vi "CRYAPI Temp Frame.vi"() -> ()   [LabVIEW 2013]
uses:
  <vilib>/Utility/miscctls.llb/LVPointTypeDef.ctl
  <vilib>/Utility/miscctls.llb/LVPositionTypeDef.ctl
  <vilib>/Utility/miscctls.llb/LVBoundsTypeDef.ctl
  <vilib>/Utility/inputDevices.llb/closeMouse.vi
  CRYMain Sub Window Global.vi
  <vilib>/Utility/inputDevices.llb/mouseAcquire.vi
panel:
  in  "StateOut":bool
  in  "IconRing":u16(ring)
  out "bTitleChange":bool
  in  "WindowNumber":i32=2
  in  "ActiveNumber":i32=2
  out "TitleName":string="Project"
  in  "PinFalse":bool
  in  "PinTrue":bool
  in  "stop":bool
  in  "InActiveClose":bool
  in  "ActiveClose":bool
  in  "nWinType":i32=2
  in  "MousePos":T1
  in  "sMsgCommand":string="Project"
  in  "nData":i32=2
  in  "FloatEvent":bool
  out "SubVI Ref":refnum<vi>
  in  "WindowName":string="Project"
  in  "DockState":bool
  in  "ActiveState":bool
  in  "ToolBarClick":bool
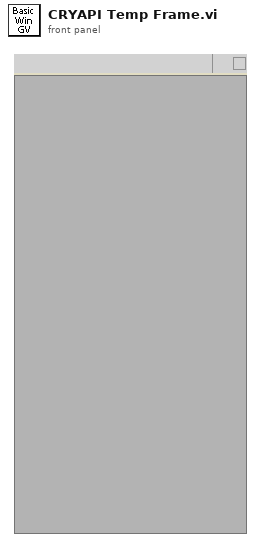
[diagram p1: front panel]
types:
  T1 = cluster{"Horizontal":i32, "Vertical":i32, "Scrolling":i32}
  T2 = typedef "LVBoundsTypeDef.ctl" = cluster{"Width":u32, "Height":u32}
  T3 = typedef "LVPositionTypeDef.ctl" = cluster{"Left":i32, "Top":i32}
  T4 = typedef "LVPointTypeDef.ctl" = cluster{"Horizontal":i16, "Vertical":i16}
  T5 = typedef "LVRectTypeDef.ctl" = cluster{"Left":i16, "Top":i16, "Right":i16, "Bottom":i16}
  T6 = cluster{"button 1":bool, "button 2":bool, "button 3":bool, "button 4":bool}
  T7 = cluster{"CLOSE_HIDE":i32, "CLOSE_CLOSE":i32, "DOCK_ENABLE":i32, "DOCK_DISABLE":i32, "FOCUS_SHOW":i32, "FOCUS_HIDE":i32}
  T8 = cluster{"nType":i32, "nParent":i32, "pVIW":refnum<vi>, "pSPW":refnum<vi>, "nTypeF":i32, "pVIF":refnum<vi>, "pSPF":refnum<vi>, "nIDSpliter":i32, "nProperty":i32, "Bound":T5, "nID":i32, "nData":i32, "sData":string, "pWVI":refnum<vi>, "sTitle":string, "cPages":cluster{"nPage":i32, "sTitle":string, "sIcon":string, "pVI":refnum<vi>, "nID":i32}[], "pTab":refnum<vi>, "nIDPages":i32[], "pSPT":refnum<vi>, "sTemp":string, "nDockID":i32, "nDockLR":i32, "sIcon":string}
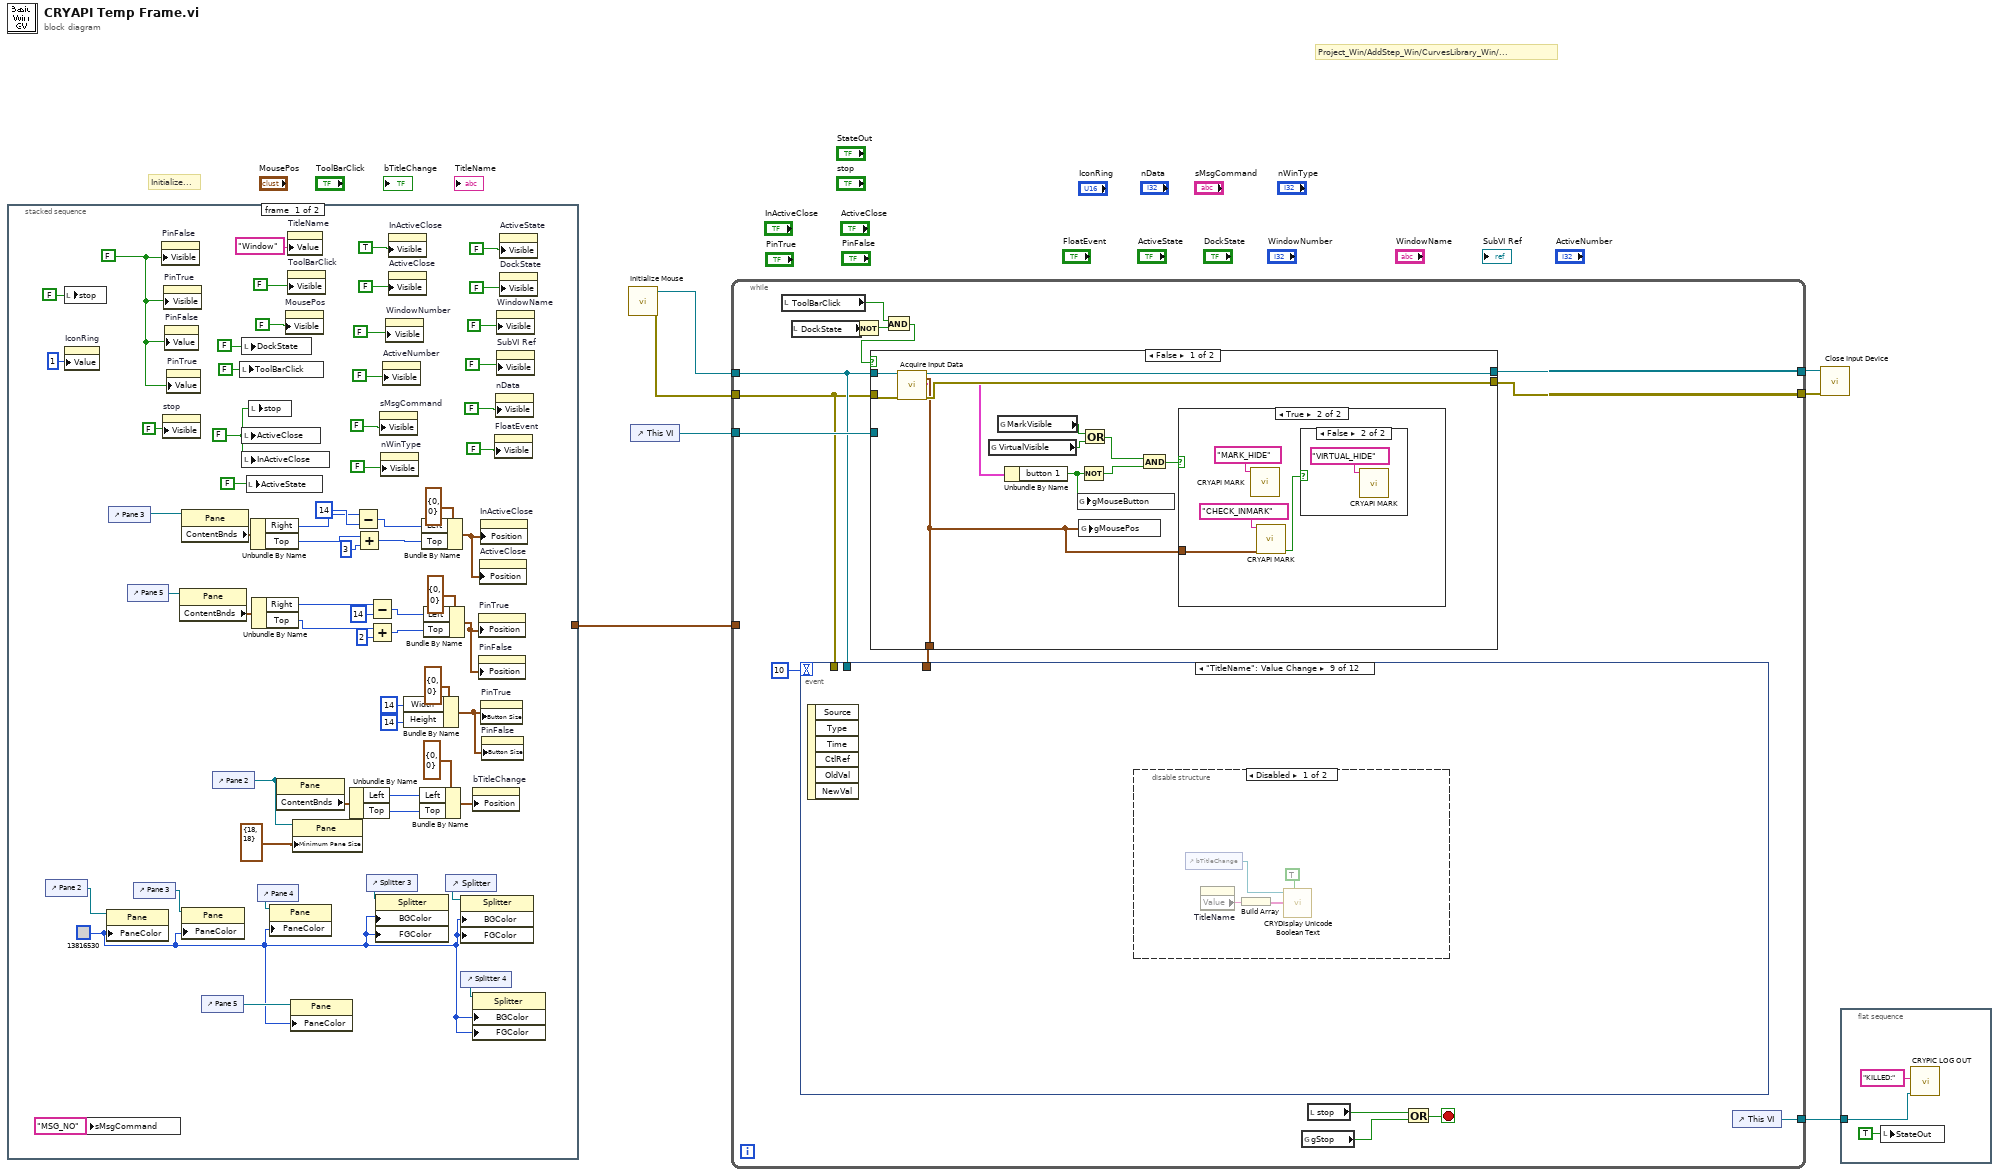
[diagram p0: block diagram]
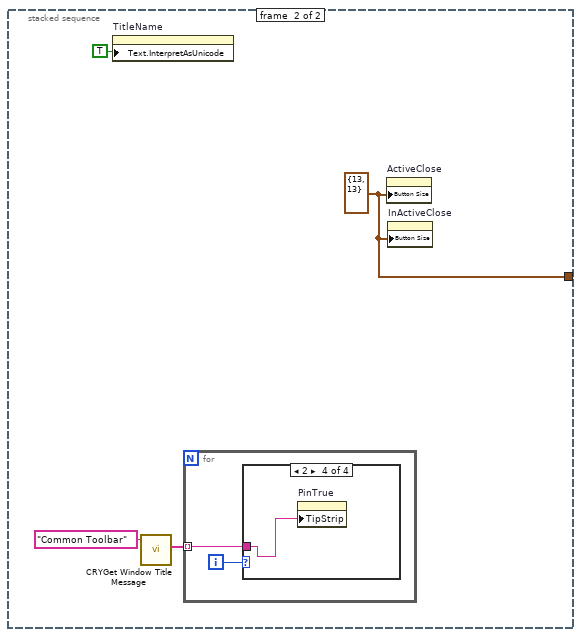
[diagram p2: hidden frame]
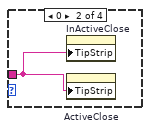
[diagram p4: hidden frame]
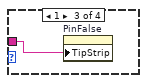
[diagram p5: hidden frame]
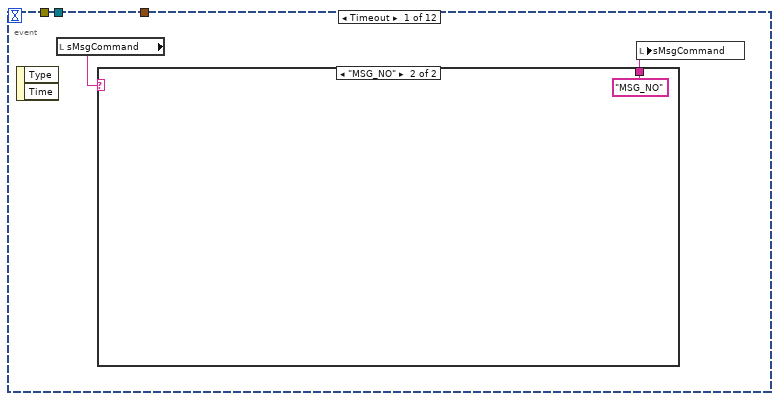
[diagram p6: hidden frame]
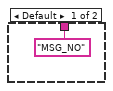
[diagram p7: hidden frame]
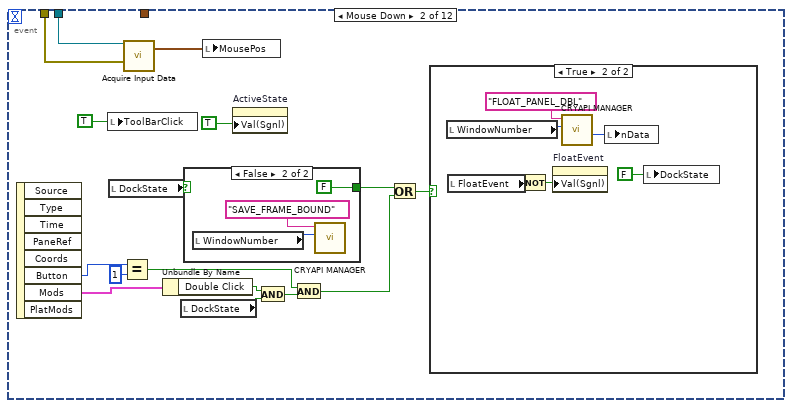
[diagram p8: hidden frame]
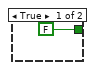
[diagram p9: hidden frame]
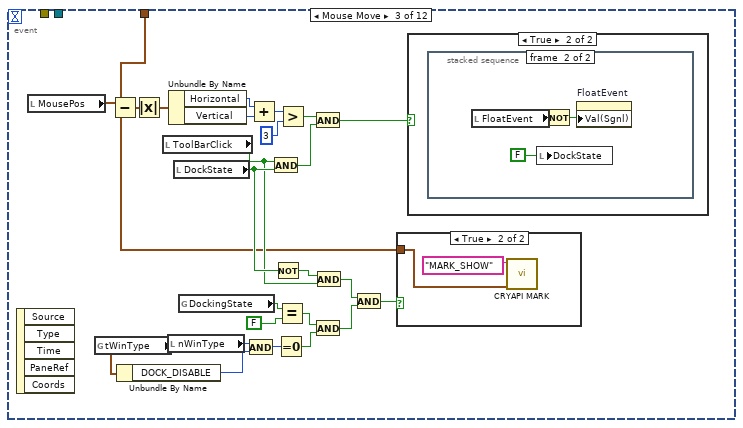
[diagram p11: hidden frame]
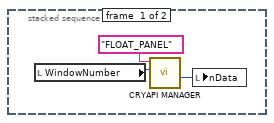
[diagram p13: hidden frame]
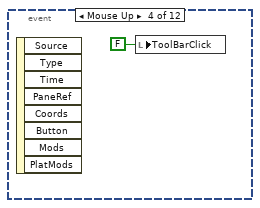
[diagram p15: hidden frame]
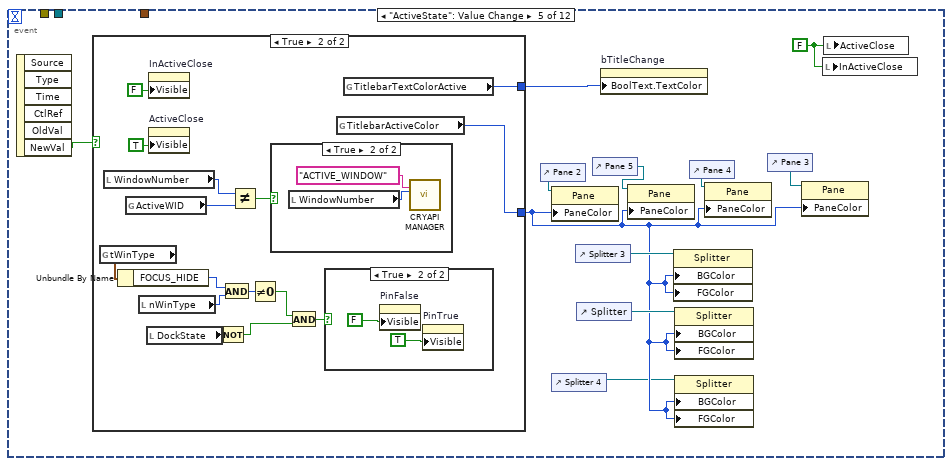
[diagram p16: hidden frame]
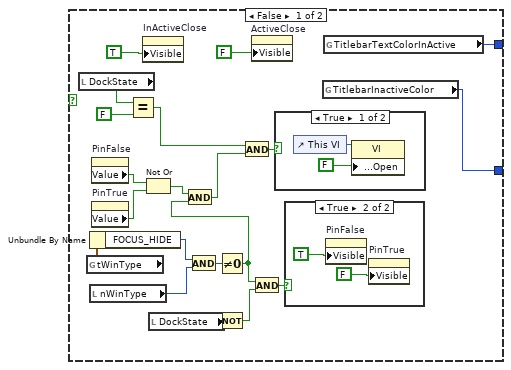
[diagram p17: hidden frame]
diagram:
  # "Project_Win/AddStep_Win/CurvesLibrary_Win/..."
  # "Initialize..."
  n1 = stacked-sequence {
    tunnel: [_ w74] -> w1
    frame #0 {
      w21 = FALSE ("Visible")
      w16 = u32 13816530
      w20 = FALSE ("Stop")
      n2 = control-ref of="Pane 2"() -> (w26:refnum<vi>)
      n3 = local write "stop"(FALSE ("stop")) -> ()
      n4 = property on="IconRing" class="Ring (strict)"("Value"=u16 1 ("Ring")) -> ()  [unwired: 2 in, 2 out]
      n5 = local write "sMsgCommand"("MSG_NO" ("sMsgCommand")) -> ()
      n6 = property class="Pane"(reference=w26, "PaneColor"=w16) -> ()  [unwired: 1 in, 2 out]
      n7 = control-ref of="Pane 3"() -> (w15:refnum<vi>)
      n8 = control-ref of="Pane 5"() -> (w8:refnum<vi>)
      n9 = control-ref of="Pane 3"() -> (w14:refnum<vi>)
      n10 = property on="PinFalse" class="Bool (strict)"("Visible"=w21) -> ()  [unwired: 2 in, 2 out]
      n11 = property on="stop" class="Bool (strict)"("Visible"=FALSE) -> ()  [unwired: 2 in, 2 out]
      n12 = property on="PinTrue" class="Bool (strict)"("Visible"=w21) -> ()  [unwired: 2 in, 2 out]
      n13 = property on="PinFalse" class="Bool (strict)"("Value"=w21) -> ()  [unwired: 2 in, 2 out]
      n14 = property on="PinTrue" class="Bool (strict)"("Value"=w21) -> ()  [unwired: 2 in, 2 out]
      n15 = property class="Pane"(reference=w8) -> ("ContentBnds"=w11:T5)  [unwired: 1 in, 2 out]
      n16 = property class="Pane"(reference=w15) -> ("ContentBnds"=w62:T5)  [unwired: 1 in, 2 out]
      n17 = property class="Pane"(reference=w14, "PaneColor"=w16) -> ()  [unwired: 1 in, 2 out]
      n18 = control-ref of="Pane 5"() -> (w18:refnum<vi>)
      n19 = control-ref of="Pane 2"() -> (w25:refnum<vi>)
      n20 = local write "ToolBarClick"(FALSE ("Click State")) -> ()
      n21 = local write "DockState"(FALSE ("DockState")) -> ()
      n22 = local write "ActiveClose"(w20) -> ()
      n23 = local write "InActiveClose"(w20) -> ()
      n24 = local write "ActiveState"(FALSE ("ActiveState")) -> ()
      n25 = local write "stop"(w20) -> ()
      n26 = Unbundle By Name(w62) -> ("Right"=w37:i16, "Top"=w32:i16)
      n27 = Unbundle By Name(w11) -> ("Right"=w10:i16, "Top"=w9:i16)
      n28 = control-ref of="Pane 4"() -> (w22:refnum<vi>)
      n29 = property class="Pane"(reference=w22, "PaneColor"=w16) -> ()  [unwired: 1 in, 2 out]
      n30 = property class="Pane"(reference=w25) -> ("ContentBnds"=w70:T5)  [unwired: 1 in, 2 out]
      n31 = property on="MousePos" class="Clust (strict)"("Visible"=FALSE) -> ()  [unwired: 2 in, 2 out]
      n32 = property on="TitleName" class="Str"("Value"="Window" ("Title Name")) -> ()  [unwired: 2 in, 2 out]
      n33 = property on="ToolBarClick" class="Bool (strict)"("Visible"=FALSE ("Click State")) -> ()  [unwired: 2 in, 2 out]
      n34 = property class="Pane"(reference=w18, "PaneColor"=w16) -> ()  [unwired: 1 in, 2 out]
      n35 = property class="Pane"(reference=w25, "Minimum Pane Size"=T4 {"Horizontal"=18, "Vertical"=18}) -> ()  [unwired: 1 in, 2 out]
      n36 = Unbundle By Name(w70) -> ("Left"=w69:i16, "Top"=w67:i16)
      n37 = Subtract(x=w37, y=i16 14) -> (x-y=w40:i16)
      n38 = Add(x=w32, y=i16 3) -> (x+y=w38:i16)
      n39 = control-ref of="Splitter 3"() -> (w56:refnum<vi>)
      n40 = Subtract(x=w10, y=i16 14) -> (x-y=w34:i16)
      n41 = Add(x=w9, y=i16 2) -> (x+y=w33:i16)
      n42 = property class="Splitter"(reference=w56, "BGColor"=w16, "FGColor"=w16) -> ()  [unwired: 1 in, 2 out]
      n43 = property on="sMsgCommand" class="Str"("Visible"=FALSE) -> ()  [unwired: 2 in, 2 out]
      n44 = property on="nWinType" class="DigNum (strict)"("Visible"=FALSE) -> ()  [unwired: 2 in, 2 out]
      n45 = property on="ActiveNumber" class="DigNum (strict)"("Visible"=FALSE) -> ()  [unwired: 2 in, 2 out]
      n46 = property on="WindowNumber" class="DigNum (strict)"("Visible"=FALSE ("ToolBar Click")) -> ()  [unwired: 2 in, 2 out]
      n47 = property on="InActiveClose" class="Bool (strict)"("Visible"=TRUE ("ToolBar Click")) -> ()  [unwired: 2 in, 2 out]
      n48 = property on="ActiveClose" class="Bool (strict)"("Visible"=FALSE ("ToolBar Click")) -> ()  [unwired: 2 in, 2 out]
      n49 = Bundle By Name(cluster=T2 {"Width"=0, "Height"=0} ("Button Size"), "Width"=u32 14, "Height"=u32 14) -> (w27:T2)
      n50 = Bundle By Name(cluster=T3 {"Left"=0, "Top"=0} ("Position"), "Left"=w69, "Top"=w67) -> (w66:T3)
      n51 = Bundle By Name(cluster=T3 {"Left"=0, "Top"=0} ("Position"), "Left"=w40, "Top"=w38) -> (w60:T3)
      n52 = Bundle By Name(cluster=T3 {"Left"=0, "Top"=0} ("Position"), "Left"=w34, "Top"=w33) -> (w31:T3)
      n53 = control-ref of="Splitter"() -> (w24:refnum<vi>)
      n54 = property class="Splitter"(reference=w24, "BGColor"=w16, "FGColor"=w16) -> ()  [unwired: 1 in, 2 out]
      n55 = control-ref of="Splitter 4"() -> (w17:refnum<vi>)
      n56 = property on="bTitleChange" class="Bool (strict)"("Position"=w66) -> ()  [unwired: 2 in, 2 out]
      n57 = property class="Splitter"(reference=w17, "BGColor"=w16, "FGColor"=w16) -> ()  [unwired: 1 in, 2 out]
      n58 = property on="PinTrue" class="Bool (strict)"("Position"=w31) -> ()  [unwired: 2 in, 2 out]
      n59 = property on="PinFalse" class="Bool (strict)"("Position"=w31) -> ()  [unwired: 2 in, 2 out]
      n60 = property on="ActiveClose" class="Bool (strict)"("Position"=w60) -> ()  [unwired: 2 in, 2 out]
      n61 = property on="InActiveClose" class="Bool (strict)"("Position"=w60) -> ()  [unwired: 2 in, 2 out]
      n62 = property on="PinTrue" class="Bool (strict)"("Button Size"=w27) -> ()  [unwired: 2 in, 2 out]
      n63 = property on="PinFalse" class="Bool (strict)"("Button Size"=w27) -> ()  [unwired: 2 in, 2 out]
      n64 = property on="FloatEvent" class="Bool (strict)"("Visible"=FALSE ("ToolBar Click")) -> ()  [unwired: 2 in, 2 out]
      n65 = property on="nData" class="DigNum (strict)"("Visible"=FALSE ("ToolBar Click")) -> ()  [unwired: 2 in, 2 out]
      n66 = property on="WindowName" class="Str"("Visible"=FALSE ("ToolBar Click")) -> ()  [unwired: 2 in, 2 out]
      n67 = property on="SubVI Ref" class="VIRef (strict)"("Visible"=FALSE ("ToolBar Click")) -> ()  [unwired: 2 in, 2 out]
      n68 = property on="ActiveState" class="Bool (strict)"("Visible"=FALSE ("ToolBar Click")) -> ()  [unwired: 2 in, 2 out]
      n69 = property on="DockState" class="Bool (strict)"("Visible"=FALSE ("ToolBar Click")) -> ()  [unwired: 2 in, 2 out]
    }
    frame #1 {
      w74 = T2 {"Width"=13, "Height"=13} ("Button Size")
      n70 = property on="TitleName" class="Str"("Text.InterpretAsUnicode"=TRUE ("Text.Interpret As Unicode")) -> ()  [unwired: 2 in, 2 out]
      n71 = call "CRYGet Window Title Message.vi"("Kind"="Common Toolbar") -> ("Tip Strip"=w72:string[])  [unwired: 5 in, 5 out]
      n72 = for {
        tunnel: w72 -> [w75] mode=indexing
        i -> [w76]
        n73 = case shown="2" w76 {
          tunnel: w75 -> [_ w77 w78 w79]
          frame Default {
          }
          frame 0 {
            n74 = property on="InActiveClose" class="Bool (strict)"("TipStrip"=w77) -> ()  [unwired: 2 in, 2 out]
            n75 = property on="ActiveClose" class="Bool (strict)"("TipStrip"=w77) -> ()  [unwired: 2 in, 2 out]
          }
          frame 1 {
            n76 = property on="PinFalse" class="Bool (strict)"("TipStrip"=w78) -> ()  [unwired: 2 in, 2 out]
          }
          frame 2 {
            n77 = property on="PinTrue" class="Bool (strict)"("TipStrip"=w79) -> ()  [unwired: 2 in, 2 out]
          }
        }
      }
      n78 = property on="ActiveClose" class="Bool (strict)"("Button Size"=w74) -> ()  [unwired: 2 in, 2 out]
      n79 = property on="InActiveClose" class="Bool (strict)"("Button Size"=w74) -> ()  [unwired: 2 in, 2 out]
    }
  }
  n80 = call <vilib>:"Initialize Mouse.vi"() -> ("error out"=w5:errorcluster, "device ID"=w4:refnum<k1>)  [unwired: 1 in, 9 out]
  n81 = control-ref of="This VI"() -> (w3:refnum<vi>)
  n82 = while {
    tunnel: w4 -> [w91]
    tunnel: w5 -> [w90]
    tunnel: [w94] -> w6
    tunnel: [w93] -> w7
    tunnel: w3 -> [w92]
    tunnel: [w83] -> w2
    tunnel: w1 -> [_]
    stop <- w82 stop-if-true
    n83 = local read "ToolBarClick"() -> (w86:bool)
    n84 = local read "DockState"() -> (w88:bool)
    n85 = Not(x=w88) -> (.not. x?=w87:bool)
    n86 = And(x=w86, y=w87) -> (x .and. y?=w85:bool)
    n87 = case shown="False" w85 {
      tunnel: w91 -> [w293 w312]
      tunnel: w90 -> [w292 w311]
      tunnel: [w290 w310] -> w94
      tunnel: [w291 w309] -> w93
      tunnel: w92 -> [_ w308]
      tunnel: [w284 w301] -> w89
      frame False {
        n88 = call-poly <vilib>:"Acquire Input Data.vi"("device ID"=w293, "error in (no error)"=w292) -> ("device ID"=w291:refnum<k1>, "axis info"=w284:T1, "button info"=w283:T6, "error out"=w290:errorcluster)  [unwired: 1 in, 13 out]
        n89 = global read "CRYMain Sub Window Global.vi" "VirtualVisible"() -> (w294:bool)
        n90 = global read "CRYMain Sub Window Global.vi" "MarkVisible"() -> (w289:bool)
        n91 = Unbundle By Name(w283) -> ("button 1"=w285:bool)
        n92 = global write "CRYMain Sub Window Global.vi" "gMouseButton"(w285) -> ()
        n93 = Not(x=w285) -> (.not. x?=w286:bool)
        n94 = global write "CRYMain Sub Window Global.vi" "gMousePos"(w284) -> ()
        n95 = Or(x=w289, y=w294) -> (x .or. y?=w287:bool)
        n96 = And(x=w287, y=w286) -> (x .and. y?=w288:bool)
        n97 = case shown="True" w288 {
          tunnel: w284 -> [_ w297]
          frame False {
          }
          frame True {
            n98 = call "CRYAPI MARK.vi"("sAction"="MARK_HIDE") -> ()  [unwired: 3 in, 7 out]
            n99 = call "CRYAPI MARK.vi"("sAction"="CHECK_INMARK", "MousePos"=w297) -> ("bResult"=w295:bool)  [unwired: 2 in, 6 out]
            n100 = case shown="False" w295 {
              frame True {
              }
              frame False {
                n101 = call "CRYAPI MARK.vi"("sAction"="VIRTUAL_HIDE") -> ()  [unwired: 3 in, 7 out]
              }
            }
          }
        }
      }
      frame True {
        n102 = call-poly <vilib>:"Acquire Input Data.vi"("device ID"=w312, "error in (no error)"=w311) -> ("device ID"=w309:refnum<k1>, "axis info"=w301:T1, "button info"=w300:T6, "error out"=w310:errorcluster)  [unwired: 1 in, 13 out]
        n103 = global read "CRYMain Sub Window Global.vi" "DockingState"() -> (w307:bool)
        n104 = Unbundle By Name(w300) -> ("button 1"=w303:bool)
        n105 = global write "CRYMain Sub Window Global.vi" "gMouseButton"(w303) -> ()
        n106 = global write "CRYMain Sub Window Global.vi" "gMousePos"(w301) -> ()
        n107 = Equal?(x=w307, y=FALSE) -> (x = y?=w304:bool)
        n108 = And(x=w304, y=w303) -> (x .and. y?=w302:bool)
        n109 = case shown="True" w302 {
          tunnel: w301 -> [_ w324]
          tunnel: w308 -> [_ w319]
          frame False {
            n110 = local write "ToolBarClick"(FALSE ("ToolBar Click")) -> ()
          }
          frame True {
            w323 = TRUE ("ToolBar Click In")
            n111 = local read "MousePos"() -> (w322:T1)
            n112 = call "CRYAPI Win Move.vi"("Mouse LButton In"=w323, "ToolBar Click In"=w323, "StartPositin In"=w322, "MousePositin In"=w324, "VI Ref In"=w319) -> ("StartPositin Out"=w320:T1, "VI Ref Out"=w318:refnum<vi>)  [unwired: 5 out]
            n113 = local write "MousePos"(w320) -> ()
            n114 = call "CRYAPI MARK.vi"("sAction"="CHECK_INTITLEBAR", "mVritual_VIRef"=w318, "MousePos"=w320) -> ()  [unwired: 1 in, 7 out]
          }
        }
        n115 = global read "CRYMain Sub Window Global.vi" "VirtualVisible"() -> (w305:bool)
        n116 = case shown="True" w305 {
          tunnel: w301 -> [_ w315]
          frame False {
          }
          frame True {
            n117 = call "CRYAPI MARK.vi"("sAction"="CHECK_INMARK", "MousePos"=w315) -> ("bResult"=w313:bool)  [unwired: 2 in, 6 out]
            n118 = case shown="False" w313 {
              frame True {
              }
              frame False {
                n119 = call "CRYAPI MARK.vi"("sAction"="VIRTUAL_HIDE") -> ()  [unwired: 3 in, 7 out]
              }
            }
          }
        }
      }
    }
    n120 = event shown="[8] \"TitleName\": Value Change" {
      selector: _ -> [_ _ _ _ _ _ _ _ _ _ _ _]
      dyn-events: _ -> [_ _ _ _ _ _ _ _ _ _ _ _]
      timeout: 10 -> [_ _ _ _ _ _ _ _ _ _ _ _]
      tunnel: w91 -> [_ w113 _ _ _ _ _ _ _ _ _ _]
      tunnel: w90 -> [_ w112 _ _ _ _ _ _ _ _ _ _]
      tunnel: w89 -> [_ _ w132 _ _ _ _ _ _ _ _ _]
      event Timeout {
        n121 = event-data() -> ()  [unwired: 3 out]
        n122 = local read "sMsgCommand"() -> (w96:string)
        n123 = case shown="\"MSG_NO\"" w96 {
          tunnel: ["MSG_NO" ("sMsgCommand") "MSG_NO" ("sMsgCommand")] -> w95
          frame Default {
          }
          frame "MSG_NO" {
          }
        }
        n124 = local write "sMsgCommand"(w95) -> ()
      }
      event Mouse Down {
        n125 = event-data() -> ("Button"=w108:u16, "Mods"=w111:cluster{"Double Click":bool, "Menu Key":bool})  [unwired: 7 out]
        n126 = local write "ToolBarClick"(TRUE ("Click State")) -> ()
        n127 = local read "DockState"() -> (w104:bool)
        n128 = Equal?(x=w108, y=u16 1) -> (x = y?=w106:bool)
        n129 = call-poly <vilib>:"Acquire Input Data.vi"("device ID"=w113, "error in (no error)"=w112) -> ("axis info"=w99:T1)  [unwired: 1 in, 16 out]
        n130 = Unbundle By Name(w111) -> ("Double Click"=w110:bool)
        n131 = local read "DockState"() -> (w109:bool)
        n132 = case shown="False" w104 {
          tunnel: [FALSE FALSE] -> w103
          frame True {
          }
          frame False {
            n133 = local read "WindowNumber"() -> (w117:i32)
            n134 = call "CRYAPI MANAGER.vi"("nData"=w117, "sAction"="SAVE_FRAME_BOUND") -> ()  [unwired: 3 in, 7 out]
          }
        }
        n135 = local write "MousePos"(w99) -> ()
        n136 = property on="ActiveState" class="Bool (strict)"("Val(Sgnl)"=TRUE ("Value (Signaling)")) -> ()  [unwired: 2 in, 2 out]
        n137 = And(x=w110, y=w109) -> (x .and. y?=w105:bool)
        n138 = And(x=w106, y=w105) -> (x .and. y?=w102:bool)
        n139 = Or(x=w103, y=w102) -> (x .or. y?=w101:bool)
        n140 = case shown="True" w101 {
          frame False {
          }
          frame True {
            n141 = local read "WindowNumber"() -> (w123:i32)
            n142 = local read "FloatEvent"() -> (w122:bool)
            n143 = Not(x=w122) -> (.not. x?=w120:bool)
            n144 = property on="FloatEvent" class="Bool (strict)"("Val(Sgnl)"=w120) -> ()  [unwired: 2 in, 2 out]
            n145 = call "CRYAPI MANAGER.vi"("nData"=w123, "sAction"="FLOAT_PANEL_DBL") -> ("nData_Out"=w119:i32)  [unwired: 3 in, 6 out]
            n146 = local write "nData"(w119) -> ()
            n147 = local write "DockState"(FALSE ("DockState")) -> ()
          }
        }
      }
      event Mouse Move {
        n148 = event-data() -> ()  [unwired: 6 out]
        n149 = local read "MousePos"() -> (w139:T1)
        n150 = global read "CRYMain Sub Window Global.vi" "tWinType"() -> (w131:T7)
        n151 = Subtract(x=w139, y=w132) -> (x-y=w142:T1)
        n152 = Unbundle By Name(w131) -> ("DOCK_DISABLE"=w130:i32)
        n153 = Absolute Value(x=w142) -> (abs(x)=w143:T1)
        n154 = local read "ToolBarClick"() -> (w134:bool)
        n155 = local read "nWinType"() -> (w129:i32)
        n156 = Unbundle By Name(w143) -> ("Horizontal"=w145:i32, "Vertical"=w144:i32)
        n157 = local read "DockState"() -> (w149:bool)
        n158 = global read "CRYMain Sub Window Global.vi" "DockingState"() -> (w137:bool)
        n159 = And(x=w129, y=w130) -> (x .and. y?=w128:i32)
        n160 = Add(x=w145, y=w144) -> (x+y=w146:i32)
        n161 = And(x=w134, y=w149) -> (x .and. y?=w140:bool)
        n162 = Not(x=w149) -> (.not. x?=w133:bool)
        n163 = Equal To 0?(x=w128) -> (x = 0?=w126:bool)
        n164 = Equal?(x=w137, y=FALSE) -> (x = y?=w127:bool)
        n165 = Greater?(x=w146, y=3) -> (0:w141:bool)
        n166 = And(x=w141, y=w140) -> (x .and. y?=w148:bool)
        n167 = And(x=w127, y=w126) -> (x .and. y?=w125:bool)
        n168 = And(x=w133, y=w134) -> (x .and. y?=w135:bool)
        n169 = And(x=w135, y=w125) -> (x .and. y?=w136:bool)
        n170 = case shown="True" w136 {
          tunnel: w132 -> [_ w156]
          frame False {
          }
          frame True {
            n171 = call "CRYAPI MARK.vi"("sAction"="MARK_SHOW", "MousePos"=w156) -> ()  [unwired: 2 in, 7 out]
          }
        }
        n172 = case shown="True" w148 {
          frame False {
          }
          frame True {
            n173 = stacked-sequence {
              frame #0 {
                n174 = local read "WindowNumber"() -> (w151:i32)
                n175 = call "CRYAPI MANAGER.vi"("nData"=w151, "sAction"="FLOAT_PANEL") -> ("nData_Out"=w150:i32)  [unwired: 3 in, 6 out]
                n176 = local write "nData"(w150) -> ()
              }
              frame #1 {
                n177 = local read "FloatEvent"() -> (w155:bool)
                n178 = local write "DockState"(FALSE ("DockState")) -> ()
                n179 = Not(x=w155) -> (.not. x?=w154:bool)
                n180 = property on="FloatEvent" class="Bool (strict)"("Val(Sgnl)"=w154) -> ()  [unwired: 2 in, 2 out]
              }
            }
          }
        }
      }
      event Mouse Up {
        n181 = event-data() -> ()  [unwired: 9 out]
        n182 = local write "ToolBarClick"(FALSE ("ToolBar Click")) -> ()
      }
      event "ActiveState": Value Change {
        w167 = FALSE ("Stop")
        n183 = event-data() -> ("NewVal"=w169:bool)  [unwired: 6 out]
        n184 = case shown="True" w169 {
          tunnel: [w170 w194] -> w160
          tunnel: [w171 w195] -> w163
          frame False {
            n185 = local read "DockState"() -> (w179:bool)
            n186 = global read "CRYMain Sub Window Global.vi" "tWinType"() -> (w187:T7)
            n187 = Unbundle By Name(w187) -> ("FOCUS_HIDE"=w184:i32)
            n188 = local read "nWinType"() -> (w185:i32)
            n189 = property on="PinFalse" class="Bool (strict)"() -> ("Value"=w182:bool)  [unwired: 2 in, 2 out]
            n190 = property on="PinTrue" class="Bool (strict)"() -> ("Value"=w183:bool)  [unwired: 2 in, 2 out]
            n191 = Equal?(x=w179, y=FALSE) -> (x = y?=w177:bool)
            n192 = property on="InActiveClose" class="Bool (strict)"("Visible"=TRUE ("ToolBar Click")) -> ()  [unwired: 2 in, 2 out]
            n193 = Not Or(1:w183, 2:w182) -> (0:w180:bool)
            n194 = local read "DockState"() -> (w173:bool)
            n195 = And(x=w184, y=w185) -> (x .and. y?=w181:i32)
            n196 = Not Equal To 0?(x=w181) -> (x != 0?=w174:bool)
            n197 = And(x=w180, y=w174) -> (x .and. y?=w176:bool)
            n198 = Not(x=w173) -> (.not. x?=w172:bool)
            n199 = And(x=w177, y=w176) -> (x .and. y?=w186:bool)
            n200 = property on="ActiveClose" class="Bool (strict)"("Visible"=FALSE ("ToolBar Click")) -> ()  [unwired: 2 in, 2 out]
            n201 = And(x=w174, y=w172) -> (x .and. y?=w175:bool)
            n202 = case shown="True" w186 {
              frame True {
                n203 = control-ref of="This VI"() -> (w193:refnum<vi>)
                n204 = property class="VI"(reference=w193, "Front Panel.Open"=FALSE ("Front Panel Window:Open")) -> ()  [unwired: 1 in, 2 out]
              }
              frame False {
              }
            }
            n205 = case shown="True" w175 {
              frame False {
              }
              frame True {
                n206 = property on="PinFalse" class="Bool (strict)"("Visible"=TRUE) -> ()  [unwired: 2 in, 2 out]
                n207 = property on="PinTrue" class="Bool (strict)"("Visible"=FALSE) -> ()  [unwired: 2 in, 2 out]
              }
            }
            n208 = global read "CRYMain Sub Window Global.vi" "TitlebarInactiveColor"() -> (w170:u32)
            n209 = global read "CRYMain Sub Window Global.vi" "TitlebarTextColorInActive"() -> (w171:u32)
          }
          frame True {
            n210 = global read "CRYMain Sub Window Global.vi" "tWinType"() -> (w204:T7)
            n211 = local read "WindowNumber"() -> (w196:i32)
            n212 = Unbundle By Name(w204) -> ("FOCUS_HIDE"=w203:i32)
            n213 = global read "CRYMain Sub Window Global.vi" "ActiveWID"() -> (w206:i32)
            n214 = local read "nWinType"() -> (w202:i32)
            n215 = local read "DockState"() -> (w201:bool)
            n216 = property on="InActiveClose" class="Bool (strict)"("Visible"=FALSE ("ToolBar Click")) -> ()  [unwired: 2 in, 2 out]
            n217 = property on="ActiveClose" class="Bool (strict)"("Visible"=TRUE ("ToolBar Click")) -> ()  [unwired: 2 in, 2 out]
            n218 = Not(x=w201) -> (.not. x?=w197:bool)
            n219 = And(x=w203, y=w202) -> (x .and. y?=w199:i32)
            n220 = Not Equal?(x=w196, y=w206) -> (x != y?=w205:bool)
            n221 = Not Equal To 0?(x=w199) -> (x != 0?=w198:bool)
            n222 = case shown="True" w205 {
              frame False {
              }
              frame True {
                n223 = local read "WindowNumber"() -> (w211:i32)
                n224 = call "CRYAPI MANAGER.vi"("nData"=w211, "sAction"="ACTIVE_WINDOW") -> ()  [unwired: 3 in, 7 out]
              }
            }
            n225 = And(x=w198, y=w197) -> (x .and. y?=w200:bool)
            n226 = case shown="True" w200 {
              frame False {
              }
              frame True {
                n227 = property on="PinFalse" class="Bool (strict)"("Visible"=FALSE) -> ()  [unwired: 2 in, 2 out]
                n228 = property on="PinTrue" class="Bool (strict)"("Visible"=TRUE) -> ()  [unwired: 2 in, 2 out]
              }
            }
            n229 = global read "CRYMain Sub Window Global.vi" "TitlebarActiveColor"() -> (w194:u32)
            n230 = global read "CRYMain Sub Window Global.vi" "TitlebarTextColorActive"() -> (w195:u32)
          }
        }
        n231 = control-ref of="Pane 2"() -> (w166:refnum<vi>)
        n232 = property class="Pane"(reference=w166, "PaneColor"=w160) -> ()  [unwired: 1 in, 2 out]
        n233 = control-ref of="Splitter 4"() -> (w159:refnum<vi>)
        n234 = control-ref of="Splitter 3"() -> (w168:refnum<vi>)
        n235 = control-ref of="Splitter"() -> (w165:refnum<vi>)
        n236 = control-ref of="Pane 5"() -> (w162:refnum<vi>)
        n237 = property on="bTitleChange" class="Bool (strict)"("BoolText.TextColor"=w163) -> ()  [unwired: 2 in, 2 out]
        n238 = property class="Pane"(reference=w162, "PaneColor"=w160) -> ()  [unwired: 1 in, 2 out]
        n239 = property class="Splitter"(reference=w168, "BGColor"=w160, "FGColor"=w160) -> ()  [unwired: 1 in, 2 out]
        n240 = property class="Splitter"(reference=w165, "BGColor"=w160, "FGColor"=w160) -> ()  [unwired: 1 in, 2 out]
        n241 = property class="Splitter"(reference=w159, "BGColor"=w160, "FGColor"=w160) -> ()  [unwired: 1 in, 2 out]
        n242 = control-ref of="Pane 4"() -> (w164:refnum<vi>)
        n243 = property class="Pane"(reference=w164, "PaneColor"=w160) -> ()  [unwired: 1 in, 2 out]
        n244 = control-ref of="Pane 3"() -> (w161:refnum<vi>)
        n245 = property class="Pane"(reference=w161, "PaneColor"=w160) -> ()  [unwired: 1 in, 2 out]
        n246 = local write "InActiveClose"(w167) -> ()
        n247 = local write "ActiveClose"(w167) -> ()
      }
      event "PinTrue", "PinFalse": Value Change {
        n248 = event-data() -> ()  [unwired: 7 out]
        n249 = local read "WindowNumber"() -> (w214:i32)
        n250 = property on="PinTrue" class="Bool (strict)"() -> ("Visible"=w217:bool)  [unwired: 2 in, 2 out]
        n251 = global read "CRYMain Sub Window Global.vi" "ActiveWID"() -> (w215:i32)
        n252 = case shown="False" w217 {
          tunnel: [w219 w220] -> w216
          frame False {
            n253 = property on="PinFalse" class="Bool (strict)"() -> ("Value"=w219:bool)  [unwired: 2 in, 2 out]
          }
          frame True {
            n254 = property on="PinTrue" class="Bool (strict)"() -> ("Value"=w220:bool)  [unwired: 2 in, 2 out]
          }
        }
        n255 = Not Equal?(x=w215, y=w214) -> (x != y?=w213:bool)
        n256 = case shown="True" w213 {
          frame False {
          }
          frame True {
            n257 = property on="ActiveState" class="Bool (strict)"("Val(Sgnl)"=TRUE ("Value (Signaling)")) -> ()  [unwired: 2 in, 2 out]
          }
        }
        n258 = property on="PinFalse" class="Bool (strict)"("Value"=w216) -> ()  [unwired: 2 in, 2 out]
        n259 = property on="PinTrue" class="Bool (strict)"("Value"=w216) -> ()  [unwired: 2 in, 2 out]
      }
      event "FloatEvent": Value Change {
        n260 = event-data() -> ()  [unwired: 7 out]
        n261 = local read "WindowNumber"() -> (w221:i32)
        n262 = local read "nData"() -> (w222:i32)
        n263 = call "CRYAPI FRAME.vi"("nData"=w221, "sAction"="GET_FRAME") -> ("tFrame_Out"=w223:T8)  [unwired: 4 in, 5 out]
        n264 = call "CRYAPI MANAGER.vi"("tFrame"=w223, "nData"=w222, "sAction"="FLOAT_FRAME") -> ()  [unwired: 2 in, 7 out]
      }
      event Pane Size {
        n265 = event-data() -> ()  [unwired: 7 out]
        n266 = control-ref of="Pane"() -> (w228:refnum<vi>)
        n267 = control-ref of="Basic Sub Panel"() -> (w226:refnum<vi>)
        n268 = property class="Pane"(reference=w228) -> ("Width"=w227:u32)  [unwired: 1 in, 2 out]
        n269 = invoke class="SubPnl" method="FitControlToPane"(reference=w226) -> ()  [unwired: 2 in, 3 out]
        n270 = flat-sequence {
          tunnel: w227 -> [w229]
          frame #0 {
            n271 = control-ref of="Splitter 3"() -> (w234:refnum<vi>)
            n272 = control-ref of="Splitter 4"() -> (w236:refnum<vi>)
            n273 = Subtract(x=w229, y=u32 40) -> (x-y=w230:u32)
            n274 = Subtract(x=w229, y=u32 20) -> (x-y=w232:u32)
            n275 = property class="Splitter"(reference=w236, "Position"=w232) -> (error out=w237:errorcluster)  [unwired: 1 in, 1 out]
            n276 = property class="Splitter"(reference=w234, "Position"=w230) -> (error out=w235:errorcluster)  [unwired: 1 in, 1 out]
            n277 = case shown="No Error" w237 {
              frame No Error {
              }
              frame Error {
              }
            }
            n278 = case shown="No Error" w235 {
              frame No Error {
              }
              frame Error {
              }
            }
            n279 = control-ref of="Splitter"() -> (w240:refnum<vi>)
            n280 = property class="Splitter"(reference=w240, "Position"=21 ("Splitter Position")) -> (error out=w238:errorcluster)  [unwired: 1 in, 1 out]
            n281 = case shown="No Error" w238 {
              frame No Error {
              }
              frame Error {
              }
            }
          }
        }
      }
      event "TitleName": Value Change {
        n282 = event-data() -> ()  [unwired: 7 out]
        n283 = disable-structure shown="Disabled" {
          frame Disabled {
            n284 = control-ref of="bTitleChange"() -> (w242:refnum<vi>)
            n285 = property on="TitleName" class="Str"() -> ("Value"=w244:string)  [unwired: 2 in, 2 out]
            n286 = Build Array(w244) -> (w243:string[])
            n287 = call "CRYDisplay Unicode Boolean Text.vi"("Interpret as Unicode (T)"=TRUE, "Boolean Texts [4]"=w243, "Boolean Reference"=w242) -> ()  [unwired: 5 in, 2 out]
          }
          frame Enabled {
          }
        }
      }
      event "InActiveClose", "ActiveClose": Value Change {
        n288 = event-data() -> ()  [unwired: 7 out]
        n289 = flat-sequence {
          frame #0 {
            w245 = "MSG_CLOSE_FRAME" ("input 1")
            w255 = FALSE ("ToolBar Click")
            n290 = local read "WindowNumber"() -> (w249:i32)
            n291 = call "CRYWindow PIC Project State Change.vi"() -> ()  [unwired: 12 in]
            n292 = call "CRYAPI FRAME.vi"("nData"=w249, "sAction"="GET_FRAME") -> ("tFrame_Out"=w268:T8)  [unwired: 4 in, 5 out]
            n293 = global read "CRYMain Sub Window Global.vi" "tWinType"() -> (w256:T7)
            n294 = Unbundle By Name(w268) -> ("nTypeF"=w262:i32, "nType"=w260:i32, "nProperty"=w258:i32)
            n295 = Unbundle By Name(w256) -> ("CLOSE_CLOSE"=w257:i32)
            n296 = local write "ToolBarClick"(w255) -> ()
            n297 = local write "ActiveClose"(w255) -> ()
            n298 = local write "InActiveClose"(w255) -> ()
            n299 = local write "DockState"(w255) -> ()
            n300 = Equal?(x=w260, y=1) -> (x = y?=w264:bool)
            n301 = Equal?(x=w262, y=0) -> (x = y?=w265:bool)
            n302 = And(x=w258, y=w257) -> (x .and. y?=w259:i32)
            n303 = Equal To 0?(x=w259) -> (x = 0?=w267:bool)
            n304 = And(x=w265, y=w264) -> (x .and. y?=w266:bool)
            n305 = And(x=w266, y=w267) -> (x .and. y?=w254:bool)
            n306 = Select(t="-HIDE", s=w254, f="-CLOSE") -> ()  [unwired: 1 out]
            n307 = Obtain Queue(name (unnamed)="CRYMAIN_ACTION" ("YAxisTitle"), element data type="" ("Action Type")) -> (queue out=w253:refnum<queue>)  [unwired: 3 in, 2 out]
            n308 = Format Into String(w245, w245, w249, 0 ("input 4")) -> (resulting string=w252:string)  [unwired: 3 in, 1 out]
            n309 = Enqueue Element(queue=w253, element=w252) -> ()  [unwired: 1 in, 4 out]
          }
        }
      }
      event Mouse Down {
        # "FRAME"
        n310 = event-data() -> ()  [unwired: 9 out]
        n311 = local read "TitleName"() -> (w272:string)
        n312 = Equal?(x=w272, y="") -> (x = y?=w270:bool)
        n313 = case shown="False" w270 {
          frame False {
            n314 = property on="ActiveState" class="Bool (strict)"("Val(Sgnl)"=TRUE ("Value (Signaling)")) -> ()  [unwired: 2 in, 2 out]
          }
          frame True {
          }
        }
      }
      event Mouse Leave {
        n315 = event-data() -> ()  [unwired: 5 out]
        n316 = local read "ToolBarClick"() -> (w275:bool)
        n317 = local read "DockState"() -> (w276:bool)
        n318 = And(x=w275, y=w276) -> (x .and. y?=w274:bool)
        n319 = case shown="True" w274 {
          frame False {
          }
          frame True {
            n320 = local read "WindowNumber"() -> (w281:i32)
            n321 = local read "FloatEvent"() -> (w280:bool)
            n322 = Not(x=w280) -> (.not. x?=w278:bool)
            n323 = property on="FloatEvent" class="Bool (strict)"("Val(Sgnl)"=w278) -> ()  [unwired: 2 in, 2 out]
            n324 = call "CRYAPI MANAGER.vi"("nData"=w281, "sAction"="FLOAT_PANEL") -> ("nData_Out"=w277:i32)  [unwired: 3 in, 6 out]
            n325 = local write "nData"(w277) -> ()
            n326 = local write "DockState"(FALSE ("DockState")) -> ()
          }
        }
      }
    }
    n327 = global read "CRYMain Sub Window Global.vi" "gStop"() -> (w84:bool)
    n328 = local read "stop"() -> (w80:bool)
    n329 = Or(x=w80, y=w84) -> (x .or. y?=w82:bool)
    n330 = control-ref of="This VI"() -> (w83:refnum<vi>)
  }
  n331 = call-poly <vilib>:"Close Input Device.vi"("error in (no error)"=w6, "device ID"=w7) -> ()  [unwired: 9 out]
  n332 = flat-sequence {
    tunnel: w2 -> [w326]
    frame #0 {
      n333 = local write "StateOut"(TRUE ("StateOut")) -> ()
      n334 = call "CRYPIC LOG OUT.vi"("pVIRef"=w326, "sData"="KILLED:") -> ()  [unwired: 10 in]
    }
  }
